vi "CSM Module - TCP Server Module(Multi-Loop Support).vi"(7 "Name(\"\" to use uuid)":string="Event CSM Tiny") -> ()   [LabVIEW 2017]
doc: "Demonstrates how to set up a basic TCP connection, send data to the specified port once a connection has been established, and terminate the connection once the data has been sent. This VI is designed to stop if the TCP connection is terminated. The data sent in this example is an array of random numbers."
uses:
  user.lib/_NEVSTOP/Communicable State Machine(CSM)/AdvanceAPI/CSM - Make String Arguments Safe.vi
  user.lib/_NEVSTOP/Communicable State Machine(CSM)/AdvanceAPI/CSM - Break Down Multiple States String.vi
  user.lib/_NEVSTOP/Communicable State Machine(CSM)/AdvanceAPI/CSM - Compact Multiple States.vi
  user.lib/_NEVSTOP/Communicable State Machine(CSM)/AdvanceAPI/CSM - Keywords.vi
  user.lib/_NEVSTOP/Communicable State Machine(CSM)/AdvanceAPI/CSM - List Modules.vi
  user.lib/_NEVSTOP/Communicable State Machine(CSM)/Communicable State Machine.lvlib
panel:
  in  "Send String":string
  out "Connected":bool
  out "TCP Received":string
  out "TCP":refnum<k5>
  out "State History":string
  # "Overview:\n\nThe sentence after polishing: \"This example demonstrates how to create a CSM module with a side loop. In some scenarios, it is much simpler to implement logic outside the CSM loop. In these cases, you can utilize the side-loop support APIs to integrate your logic with the CSM loop and form a submodule. \n\nA simple TCP server submodule is created in this example, which is intuitive and takes advantage of CSM as the interface.\n\nInstructions::\n\n1. Run this VI.\n2. Run the slightly modified Simple TCP - Client.vi, which is based on the LabVIEW example.\n3. Modify the String control on both this front panel and the client, and observe the log information.\n4. You can restart Simple TCP - Client.vi to view the logs."
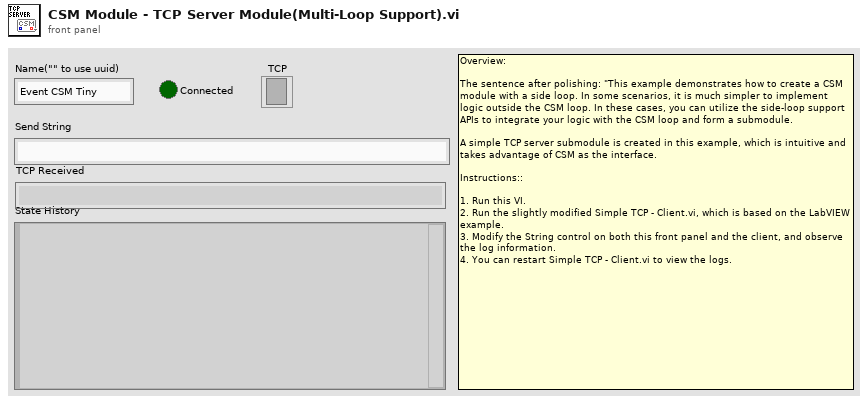
[diagram p1: front panel]
types:
  T1 = enum32{"Invalid", "Standard", "Closed", "Hidden", "Minimized", "Maximized"}
  T2 = enum32{"invalid app kind", "Development System", "Run Time System", "Student Edition", "Embedded LabVIEW", "Evaluation", "Custom"}
  T3 = typedef "Communicable State Machine.lvlib/_CSM_Response Source Message.ctl" = cluster{"‘State":string, "’Arguments":string, "’Error":errorcluster}
  T4 = cluster{"Current VI Reference":refnum<vi>, "Close Panel on Exit?":bool}
  T5 = cluster{"Core":cluster{"Current VI Reference":refnum<vi>, "Close Panel on Exit?":bool}, "Your Boolean data":bool, "Your string data":string}
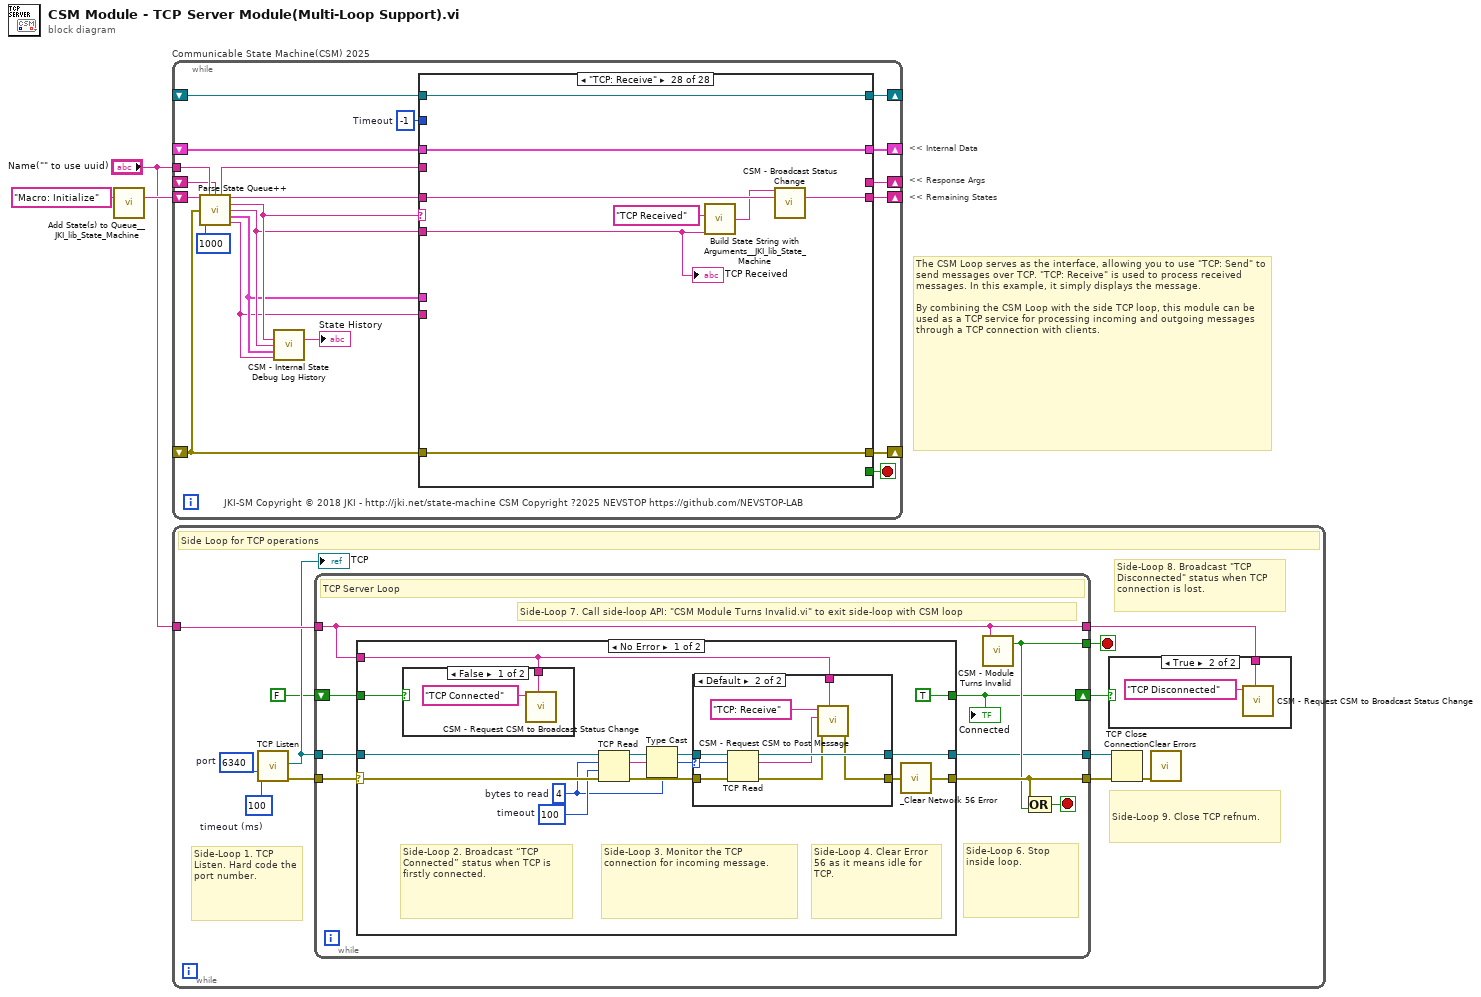
[diagram p0: block diagram]
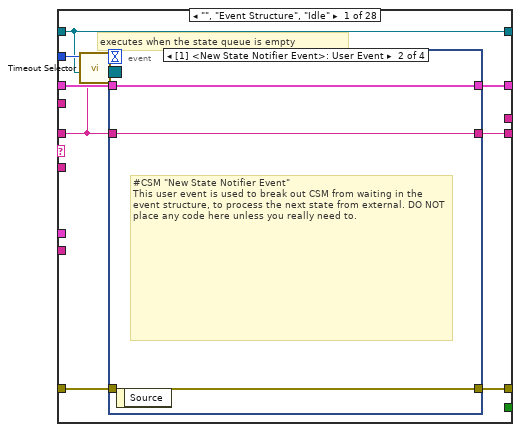
[diagram p2: hidden frame]
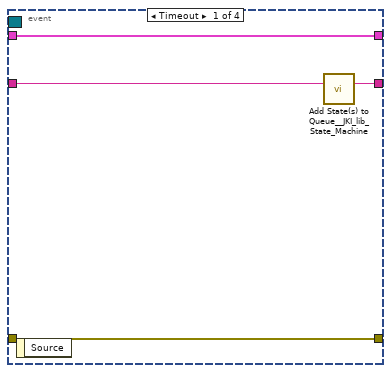
[diagram p3: hidden frame]
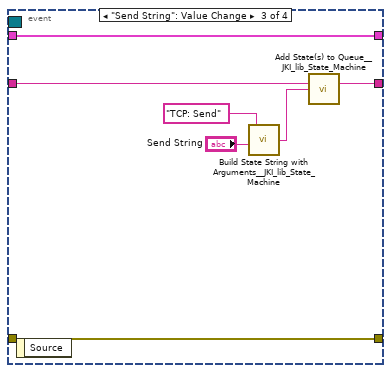
[diagram p4: hidden frame]
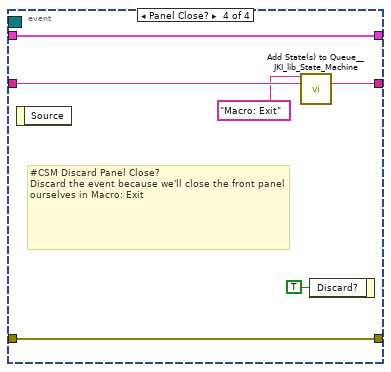
[diagram p5: hidden frame]
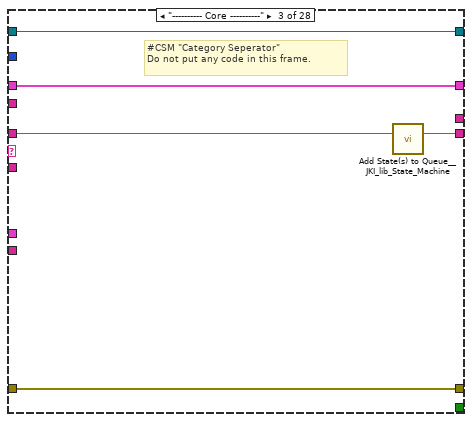
[diagram p7: hidden frame]
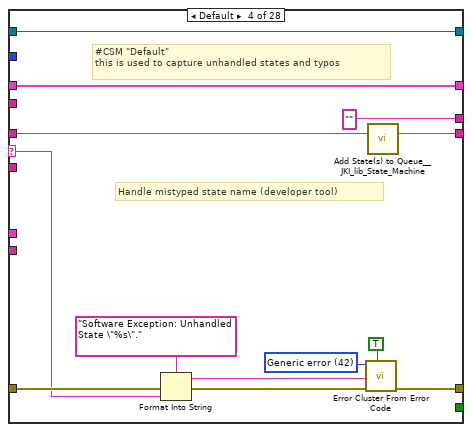
[diagram p8: hidden frame]
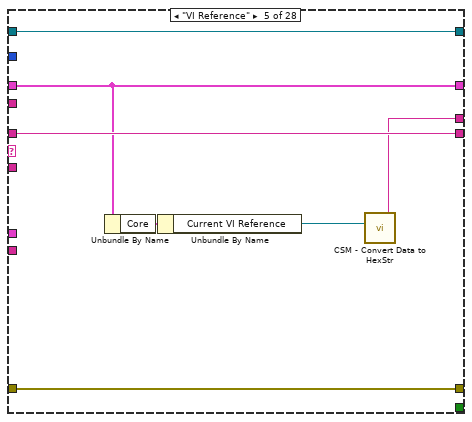
[diagram p9: hidden frame]
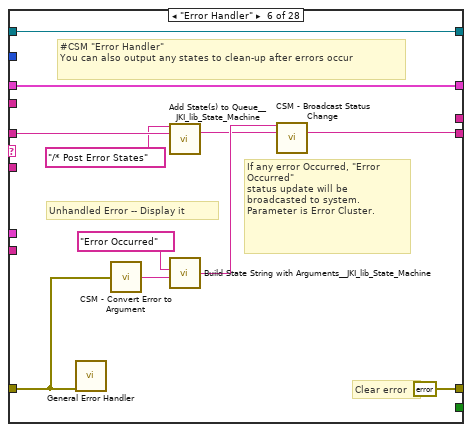
[diagram p10: hidden frame]
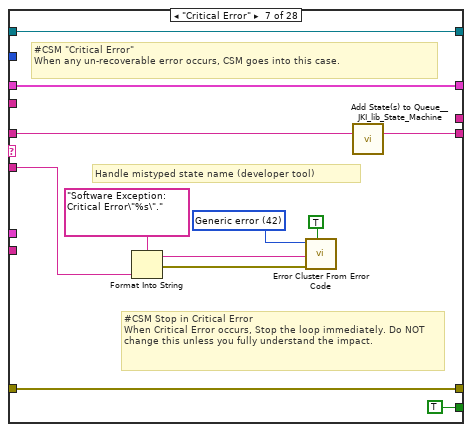
[diagram p11: hidden frame]
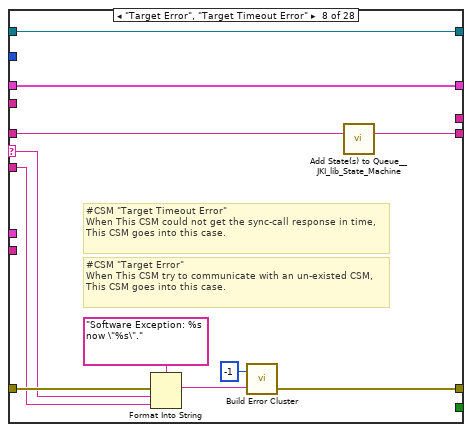
[diagram p12: hidden frame]
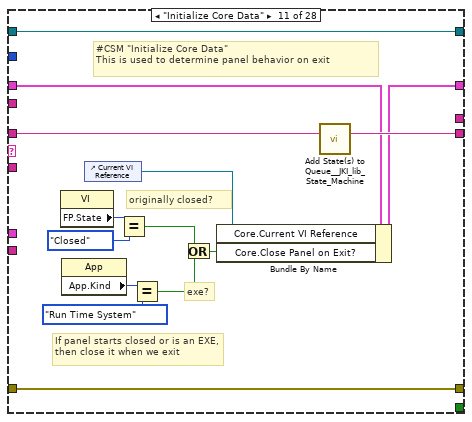
[diagram p15: hidden frame]
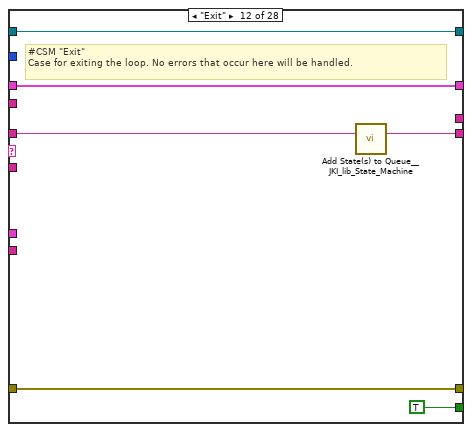
[diagram p16: hidden frame]
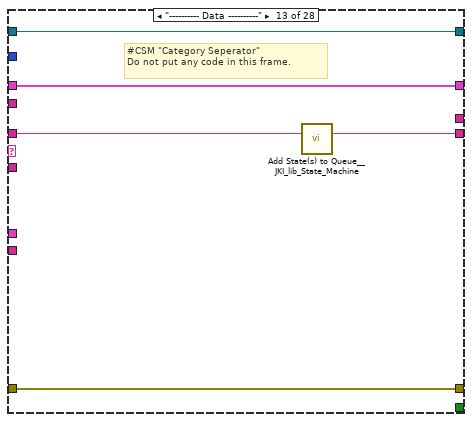
[diagram p17: hidden frame]
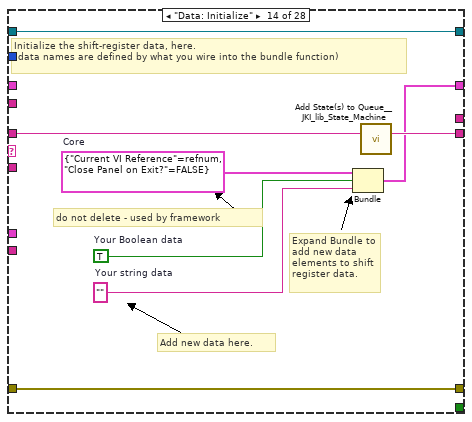
[diagram p18: hidden frame]
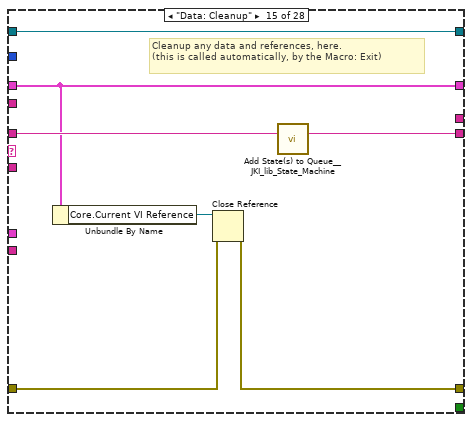
[diagram p19: hidden frame]
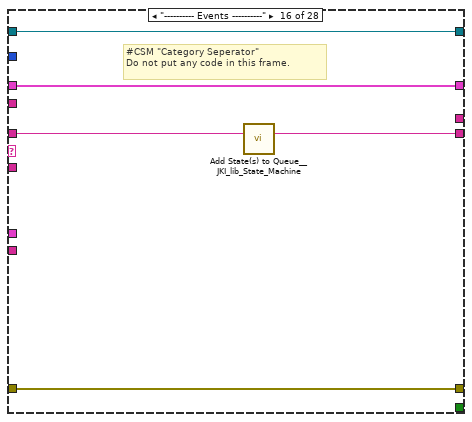
[diagram p20: hidden frame]
diagram:
  # "The CSM Loop serves as the interface, allowing you to use \"TCP: Send\" to send messages over TCP. \"TCP: Receive\" is used to process received messages. In this example, it simply displays the message. \n\nBy combining the CSM Loop with the side TCP loop, this module can be used as a TCP service for processing incoming and outgoing messages through a TCP connection with clients."
  # "<< Internal Data"
  # "<< Response Args"
  # "<< Remaining States"
  n1 = call <vilib>:"Add State(s) to Queue__JKI_lib_State_Machine.vi"("State(s) in (\"\")"="Macro: Initialize") -> ("States Out"=w2:string)  [unwired: 14 in]
  n2 = while "Communicable State Machine(CSM) 2025" {
    shift-right: [w19] -> _
    shift-left: _ -> [w18]
    shift-right: [w22] -> _
    shift-left: _ -> [w16]
    shift-right: [w21] -> _
    shift-left: w2 -> [w23]
    tunnel: "Name(\"\" to use uuid)" -> [w11]
    shift-right: [w14] -> _
    shift-left: _ -> [w5]
    shift-right: [w13] -> _
    shift-left: _ -> [w12]
    stop <- w20 stop-if-true
    w17 = -1  # Timeout
    # "JKI-SM Copyright © 2018 JKI - http://jki.net/state-machine CSM Copyright ?2025 NEVSTOP https://github.com/NEVSTOP-LAB"
    n3 = call "Parse State Queue++.vi"("State Queue"=w23, "Name(\"\" to use uuid)"=w11, "Response Arguments"=w5, "Previous Error"=w16, "Response Timeout(-2 use global Settings)"=1000 ("Response Timeout(1000ms)")) -> ("Name Used"=w6:string, "Remaining States"=w24:string, "Current State"=w10:string, "Arguments"=w9:string, ">> Response Source Message >>"=w8:T3, ">> Source CSM >>"=w7:string)  [unwired: 5 in]
    n4 = call "CSM - Internal State Debug Log History.vi"("State"=w10, "Arguments (\"\")"=w9, ">> Response Source Message >>"=w8, "Source (\"\")"=w7) -> ("Debug Log"=→"State History":string)  [unwired: 11 in]
    n5 = case shown="\"TCP: Receive\"" w10 {
      selector: w10 -> [_ _ _ w65 _ _ _ w109 _ _ _ _ _ _ _ _ _ _ _ _ _ _ _ _ _ _ _ _]
      tunnel: w24 -> [w25 w56 w62 w69 w81 w93 w103 w111 w119 w123 w138 w144 w149 w157 w164 w169 w176 w180 w186 w191 w198 w214 w284 w290 w301 w304 w315 w322]
      tunnel: w9 -> [_ _ _ _ _ _ w96 w110 _ _ _ _ _ _ _ _ _ _ _ _ w193 w208 _ _ _ _ w306 w317]
      tunnel: w18 -> [w32 w55 w59 w67 w80 w91 w104 w113 w118 w122 w131 w142 w146 _ w159 w166 w175 w179 w183 w189 w196 w210 w281 w287 w298 w303 w314 w321]
      tunnel: [w31 w57 w60 w71 w82 errorcluster {"status"=FALSE, "code"=0, "source"=""} ("error out") w105 w107 w120 w124 w135 w141 w147 w154 w160 w167 w170 w178 w184 w188 w194 w211 w282 w288 w299 w305 w307 w323] -> w22
      tunnel: w16 -> [w30 w57 w60 w70 w82 w83 w105 w115 w120 w124 w135 w141 w147 w154 w161 w167 _ w181 w184 w188 w195 w212 w282 w288 w299 w305 _ w323]
      tunnel: [w33 w56 w61 w68 w81 w84 w102 w114 w119 w123 w137 w143 w148 w156 w163 w168 w176 w180 w185 w190 w197 w213 w283 w289 w300 w304 w315 w319] -> w21
      tunnel: [_ _ _ _ _ _ TRUE _ _ _ _ TRUE _ _ _ _ _ _ _ _ _ _ _ _ _ _ _ _] -> w20
      tunnel: [w29 w55 w59 w67 w80 w91 w104 w113 w118 w122 w136 w142 w146 w155 w159 w166 w175 w179 w183 w189 w196 w210 w281 w287 w298 w303 w314 w321] -> w19
      tunnel: w17 -> [w28 _ _ _ _ _ _ _ _ _ _ _ _ _ _ _ _ _ _ _ _ _ _ _ _ _ _ _]
      tunnel: w7 -> [_ _ _ _ _ _ _ _ _ _ _ _ _ _ _ _ _ _ _ _ _ _ _ _ _ _ _ _]
      tunnel: w8 -> [_ _ _ _ _ _ _ _ _ _ _ _ _ _ _ _ _ _ _ _ _ _ _ _ _ _ _ _]
      tunnel: [_ _ _ "" w76 _ _ _ _ _ _ _ _ _ _ _ _ _ _ _ _ _ _ _ _ _ _ _] -> w14
      tunnel: [w27 w54 w58 w63 w79 w89 w94 w112 w117 w121 w125 w139 w145 w150 w158 w165 w174 w177 w182 w187 w192 w207 w280 w285 w291 w302 w313 w320] -> w13
      tunnel: w12 -> [w27 w54 w58 w63 w79 w89 w94 w112 w117 w121 w125 w139 w145 w150 w158 w165 _ w177 w182 w187 w192 w207 w280 w285 w291 w302 w313 w320]
      tunnel: w6 -> [_ _ _ _ _ _ _ _ _ _ _ _ _ _ _ _ w173 _ _ _ _ _ _ _ _ _ _ _]
      frame "", "Event Structure", "Idle" {
        # "executes when the state queue is empty"
        n6 = call "Timeout Selector.vi"("Remaining States"=w25, "Timeout Expected"=w28) -> ("Timeout"=w26:i32)  [unwired: 5 in]
        n7 = event shown="[1] <New State Notifier Event>: User Event" {
          selector: w27 -> [_ _ _ _]
          dyn-events: _ -> [_ _ _ _]
          timeout: w26 -> [_ _ _ _]
          tunnel: w25 -> [w37 w39 w45 w53]
          tunnel: [w36 w39 w44 w52] -> w33
          tunnel: w32 -> [w34 w40 w46 w50]
          tunnel: [w35 w38 w47 w51] -> w31
          tunnel: w30 -> [w35 w38 w47 w51]
          tunnel: [w34 w40 w46 w50] -> w29
          event Timeout {
            n8 = event-data() -> ()  [unwired: 1 in, 1 out]
            n9 = call <vilib>:"Add State(s) to Queue__JKI_lib_State_Machine.vi"("State(s) in (\"\")"=w37) -> ("States Out"=w36:string)  [unwired: 14 in]
          }
          event User Event {
            # "#CSM \"New State Notifier Event\"\nThis user event is used to break out CSM from waiting in the event structure, to process the next state from external. DO NOT place any code here unless you really need to."
            n10 = event-data() -> ()  [unwired: 1 in, 1 out]
          }
          event "Send String": Value Change {
            n11 = event-data() -> ()  [unwired: 1 in, 1 out]
            n12 = call <vilib>:"Build State String with Arguments__JKI_lib_State_Machine.vi"("Arguments (\"\")"="Send String", "State"="TCP: Send") -> ("State with Arguments"=w42:string)  [unwired: 4 in]
            n13 = call <vilib>:"Add State(s) to Queue__JKI_lib_State_Machine.vi"("State(s) in (\"\")"=w45, "State(s) at Back (\"\")"=w42) -> ("States Out"=w44:string)  [unwired: 13 in]
          }
          event Panel Close? {
            # "#CSM Discard Panel Close?\nDiscard the event because we'll close the front panel ourselves in Macro: Exit"
            n14 = event-data() -> ()  [unwired: 1 in, 1 out]
            n15 = call <vilib>:"Add State(s) to Queue__JKI_lib_State_Machine.vi"("State(s) in Front (\"\")"="Macro: Exit", "State(s) in (\"\")"=w53) -> ("States Out"=w52:string)  [unwired: 13 in]
            n16 = event-data("Discard?"=TRUE) -> ()  [unwired: 1 in, 1 out]
          }
        }
      }
      frame "CSM Documentation" {
        # "#CSM README FIRST\n\nCSM is a LabVIEW application framework that builds upon JKI State Machine (JKISM). It follows the pattern of JKISM and extends the keywords to describe message communication between CSM modules, including concepts such as Sync-Message, Async-Message, Subscription/Unsubscription of status - essential elements for creating reusable code modules. For more information, please visit the CSM wiki: https://github.com/NEVSTOP-LAB/JKI-State-Machine-Plus-Plus/wiki\n\nFor instructions on JKI State Machine, visit: http://jki.net/state-machine/\nFor information about CSM, visit: https://github.com/NEVSTOP-LAB"
        # "#CSM \"Documentation\"\nCase for holding CSM Documenation"
      }
      frame "---------- Core ----------" {
        # "#CSM \"Category Seperator\"\nDo not put any code in this frame."
        n17 = call <vilib>:"Add State(s) to Queue__JKI_lib_State_Machine.vi"("State(s) in (\"\")"=w62) -> ("States Out"=w61:string)  [unwired: 14 in]
      }
      frame Default {
        w74 = 42 items=["No error", "Argument error", "Memory is full", "Out of zone", "End of file", "File already open", "Generic file I/O error", "File not found", "File permission error", "Disk is full", "Duplicate path", "Too many files open", "System feature not enabled", "Resource file not found", "Cannot add resource", "Resource not found", "Image not found", "Image memory error", "Pen does not exist", "Config type invalid", "Config token not found", "Config parse error", "Config memory error", "Bad external code format", "Bad external code offset", "External code not present", "Null window", "Destroy window error", "Null menu", "Print aborted", "Bad print record", "Print driver error", "Windows error during printing", "Memory error during printing", "Print dialog error", "Generic print error", "Invalid device refnum", "Device not found", "Device parameter error", "Device unit error", "Cannot open device", "Device call aborted", "Generic error", "Cancelled by user", "Object ID too low", "Object ID too high", "Object not in heap", "Unknown heap", "Unknown object (invalid DefProc)", "Unknown object (DefProc not in table)", "Message out of range", "Invalid (null) method", "Unknown message", "Manager call not supported", "Bad address", "Network operation in progress", "Network operation timed out", "Connection is busy", "Network attribute not supported", "Network error", "Address in use", "System out of memory", "Connection aborted", "Connection refused", "Not connected", "Already connected", "Connection closed", "Initialization error (interapplication manager)", "Bad occurrence", "Wait on unbound occurrence handler", "Occurrence queue overflow", "Datalog type conflict", "Unused", "Unrecognized type (interapplication manager)", "Memory corrupt", "Failed to make temporary DLL", "Old CIN version", "Drag socket not found", "Failed to load drop-object", "Failed to register OLE object", "Failed to release OLE object", "Format specifier type mismatch", "Unknown format specifier", "Too few format specifiers", "Too many format specifiers", "Scan failed", "Newer CIN version", "Error converting to variant", "Runtime menu error", "Password tampered", "Variant attribute not found", "Incompatible variant data type", "Event data is not available", "Event Store is not present", "Occurrence is not found", "Event Queue is not created", "Event info is not available", "Refnum passed is NULL", "Error retrieving Class GUID", "Error retrieving CoClass GUID", "Error retrieving TypeLib GUID.", "Bad built application magic bytes.", "Specific driver is different from the specific driver associated with the Logical Name.", "There is no session opened to the class driver.", "Max Error", "MAX - Error with config objects", "MAX - Error loading configuration", "MAX - Group not supported"]
        # "#CSM \"Default\"\nthis is used to capture unhandled states and typos"
        # "Handle mistyped state name (developer tool)"
        n18 = Format Into String(format string="Software Exception: Unhandled State \"%s\"." ("message"), error in=w70, w65) -> (resulting string=w73:string, error out=w72:errorcluster)  [unwired: 1 in]
        n19 = call <vilib>:"Error Cluster From Error Code.vi"("show call chain? (False)"=TRUE, "error in (no error)"=w72, "error message (\"\")"=w73, "error code (0)"=w74) -> ("error out"=w71:errorcluster)  [unwired: 5 in]
        n20 = call <vilib>:"Add State(s) to Queue__JKI_lib_State_Machine.vi"("State(s) in (\"\")"=w69) -> ("States Out"=w68:string)  [unwired: 14 in]
      }
      frame "VI Reference" {
        n21 = Unbundle By Name(w80) -> ("Core"=w78:T4)
        n22 = Unbundle By Name(w78) -> ("Current VI Reference"=w77:refnum<vi>)
        n23 = call "CSM - Convert Data to HexStr.vi"("Variant"=w77) -> ("HEX String (0-9,A-F)"=w76:string)  [unwired: 8 in]
      }
      frame "Error Handler" {
        # "#CSM \"Error Handler\"\nYou can also output any states to clean-up after errors occur"
        # "If any error Occurred, \"Error Occurred\" \nstatus update will be broadcasted to system.\nParameter is Error Cluster."
        # "Unhandled Error -- Display it"
        # "Clear error"
        n24 = call <vilib>:"General Error Handler.vi"("error in (no error)"=w83) -> ()  [unwired: 10 in, 5 out]
        n25 = call "CSM - Convert Error to Argument.vi"("error"=w83) -> ("Argument"=w87:string)  [unwired: 4 in]
        n26 = call <vilib>:"Add State(s) to Queue__JKI_lib_State_Machine.vi"("State(s) in Front (\"\")"="/* Post Error States", "State(s) in (\"\")"=w93) -> ("States Out"=w85:string)  [unwired: 13 in]
        n27 = call <vilib>:"Build State String with Arguments__JKI_lib_State_Machine.vi"("Arguments (\"\")"=w87, "State"="Error Occurred" ("Status with Arguments")) -> ("State with Arguments"=w86:string)  [unwired: 4 in]
        n28 = call "CSM - Broadcast Status Change.vi"("Status with Arguments"=w86, "State Queue"=w85) -> ("Remaining States"=w84:string)  [unwired: 13 in]
      }
      frame "Critical Error" {
        w100 = 42 items=["No error", "Argument error", "Memory is full", "Out of zone", "End of file", "File already open", "Generic file I/O error", "File not found", "File permission error", "Disk is full", "Duplicate path", "Too many files open", "System feature not enabled", "Resource file not found", "Cannot add resource", "Resource not found", "Image not found", "Image memory error", "Pen does not exist", "Config type invalid", "Config token not found", "Config parse error", "Config memory error", "Bad external code format", "Bad external code offset", "External code not present", "Null window", "Destroy window error", "Null menu", "Print aborted", "Bad print record", "Print driver error", "Windows error during printing", "Memory error during printing", "Print dialog error", "Generic print error", "Invalid device refnum", "Device not found", "Device parameter error", "Device unit error", "Cannot open device", "Device call aborted", "Generic error", "Cancelled by user", "Object ID too low", "Object ID too high", "Object not in heap", "Unknown heap", "Unknown object (invalid DefProc)", "Unknown object (DefProc not in table)", "Message out of range", "Invalid (null) method", "Unknown message", "Manager call not supported", "Bad address", "Network operation in progress", "Network operation timed out", "Connection is busy", "Network attribute not supported", "Network error", "Address in use", "System out of memory", "Connection aborted", "Connection refused", "Not connected", "Already connected", "Connection closed", "Initialization error (interapplication manager)", "Bad occurrence", "Wait on unbound occurrence handler", "Occurrence queue overflow", "Datalog type conflict", "Unused", "Unrecognized type (interapplication manager)", "Memory corrupt", "Failed to make temporary DLL", "Old CIN version", "Drag socket not found", "Failed to load drop-object", "Failed to register OLE object", "Failed to release OLE object", "Format specifier type mismatch", "Unknown format specifier", "Too few format specifiers", "Too many format specifiers", "Scan failed", "Newer CIN version", "Error converting to variant", "Runtime menu error", "Password tampered", "Variant attribute not found", "Incompatible variant data type", "Event data is not available", "Event Store is not present", "Occurrence is not found", "Event Queue is not created", "Event info is not available", "Refnum passed is NULL", "Error retrieving Class GUID", "Error retrieving CoClass GUID", "Error retrieving TypeLib GUID.", "Bad built application magic bytes.", "Specific driver is different from the specific driver associated with the Logical Name.", "There is no session opened to the class driver.", "Max Error", "MAX - Error with config objects", "MAX - Error loading configuration", "MAX - Group not supported"]
        # "#CSM Stop in Critical Error\nWhen Critical Error occurs, Stop the loop immediately. Do NOT change this unless you fully understand the impact."
        # "#CSM \"Critical Error\"\nWhen any un-recoverable error occurs, CSM goes into this case."
        # "Handle mistyped state name (developer tool)"
        n29 = Format Into String(format string="Software Exception: Critical Error\"%s\"." ("message"), w96) -> (resulting string=w99:string, error out=w98:errorcluster)  [unwired: 2 in]
        n30 = call <vilib>:"Error Cluster From Error Code.vi"("show call chain? (False)"=TRUE, "error in (no error)"=w98, "error message (\"\")"=w99, "error code (0)"=w100) -> ()  [unwired: 5 in, 1 out]
        n31 = call <vilib>:"Add State(s) to Queue__JKI_lib_State_Machine.vi"("State(s) in (\"\")"=w103) -> ("States Out"=w102:string)  [unwired: 14 in]
      }
      frame "Target Error", "Target Timeout Error" {
        # "#CSM \"Target Error\"\nWhen This CSM try to communicate with an un-existed CSM, This CSM goes into this case."
        # "#CSM \"Target Timeout Error\"\nWhen This CSM could not get the sync-call response in time, This CSM goes into this case."
        n32 = Format Into String(format string="Software Exception: %s now \"%s\"." ("message"), error in=w115, w109, w110) -> (resulting string=w108:string)  [unwired: 1 in, 1 out]
        n33 = call "Build Error Cluster.vi"("String to Prepend to source (\"\")"=w108, "code"=-1) -> ("error out"=w107:errorcluster)
        n34 = call <vilib>:"Add State(s) to Queue__JKI_lib_State_Machine.vi"("State(s) in (\"\")"=w111) -> ("States Out"=w114:string)  [unwired: 14 in]
      }
      frame "Async Response", "Response" {
        # "#CSM Response Comments\nAfter Message is executed, CSM goes to this state for receive the response.\n    For Async Message(->), \"Async Response\" is used. This CSM will goes to \"Async Message Posted\" immediately and receive the \"Async Response\" after the callee finishes the message.\n    For Sync Message(@),  This CSM will wait until the message is done and immediately goes to \"Response\""
        # "#CSM \"Async Response\"\nHandle Async-call Response (\"Async Response\" for ->)"
        # "#CSM \"Response\"\nHandle Sync-call Response (\"Response\" for -@)"
      }
      frame "Async Message Posted" {
        # "#CSM \"Async Message Posted\"\nAfter Async Message is posted (-> or ->| ), CSM goes to this state for post-action.\nYou can use Argument - State to tell which Async Message is called."
      }
      frame "Initialize Core Data" {
        # "#CSM \"Initialize Core Data\"\nThis is used to determine panel behavior on exit"
        # "originally closed?"
        # "exe?"
        # "If panel starts closed or is an EXE, then close it when we exit"
        n35 = property class="VI"() -> ("FP.State"=w128:T1)  [unwired: 2 in, 2 out]
        n36 = property class="App"() -> ("App.Kind"=w134:T2)  [unwired: 2 in, 2 out]
        n37 = control-ref of="Current VI Reference"() -> (w129:refnum<vi>)
        n38 = Equal?(x=w128, y=T1."Closed" ("Front Panel Window:State")) -> (x = y?=w126:bool)
        n39 = Equal?(x=w134, y=T2."Run Time System" ("Application:Kind")) -> (x = y?=w132:bool)
        n40 = Or(x=w126, y=w132) -> (x .or. y?=w130:bool)
        n41 = Bundle By Name(cluster=w131, "Core.Current VI Reference"=w129, "Core.Close Panel on Exit?"=w130) -> (w136:T5)
        n42 = call <vilib>:"Add State(s) to Queue__JKI_lib_State_Machine.vi"("State(s) in (\"\")"=w138) -> ("States Out"=w137:string)  [unwired: 14 in]
      }
      frame "Exit" {
        # "#CSM \"Exit\"\nCase for exiting the loop. No errors that occur here will be handled."
        n43 = call <vilib>:"Add State(s) to Queue__JKI_lib_State_Machine.vi"("State(s) in (\"\")"=w144) -> ("States Out"=w143:string)  [unwired: 14 in]
      }
      frame "---------- Data ----------" {
        # "#CSM \"Category Seperator\"\nDo not put any code in this frame."
        n44 = call <vilib>:"Add State(s) to Queue__JKI_lib_State_Machine.vi"("State(s) in (\"\")"=w149) -> ("States Out"=w148:string)  [unwired: 14 in]
      }
      frame "Data: Initialize" {
        w151 = T4 {"Current VI Reference"=refnum, "Close Panel on Exit?"=FALSE}  # Core
        w153 = TRUE  # Your Boolean data
        w152 = ""  # Your string data
        # "do not delete - used by framework"
        # "Expand Bundle to add new data elements to shift register data."
        # "Add new data here."
        # "Initialize the shift-register data, here.\n(data names are defined by what you wire into the bundle function)"
        n45 = Bundle("Core"=w151, "Your Boolean data"=w153, "Your string data"=w152) -> (w155:T5)  [unwired: 1 in]
        n46 = call <vilib>:"Add State(s) to Queue__JKI_lib_State_Machine.vi"("State(s) in (\"\")"=w157) -> ("States Out"=w156:string)  [unwired: 14 in]
      }
      frame "Data: Cleanup" {
        # "Cleanup any data and references, here.\n(this is called automatically, by the Macro: Exit)"
        n47 = Unbundle By Name(w159) -> ("Core.Current VI Reference"=w162:refnum<vi>)
        n48 = Close Reference(reference=w162, error in (no error)=w161) -> (error out=w160:errorcluster)
        n49 = call <vilib>:"Add State(s) to Queue__JKI_lib_State_Machine.vi"("State(s) in (\"\")"=w164) -> ("States Out"=w163:string)  [unwired: 14 in]
      }
      frame "---------- Events ----------" {
        # "#CSM \"Category Seperator\"\nDo not put any code in this frame."
        n50 = call <vilib>:"Add State(s) to Queue__JKI_lib_State_Machine.vi"("State(s) in (\"\")"=w169) -> ("States Out"=w168:string)  [unwired: 14 in]
      }
      frame "Events: Register" {
        # "#CSM \"Events: Register\"\nRegister user event. New Message Event is registered to break CSM waiting in event structure by default."
        # "#CSM Register New Message Event\nRegister message event to break Waiting in Event structure."
        n51 = call "CSM - Get New State Notifier Event.vi"("Name(\"\" to use uuid) in"=w173) -> ("Error out"=w171:errorcluster, "New State Notifier Event"=w172:refnum<user-event>)  [unwired: 9 in]
        n52 = register-events(error in=w171, w172) -> (reference out=w174:refnum<event-registration>, error out=w170:errorcluster)  [unwired: 1 in]
      }
      frame "Events: Unregister" {
        # "#CSM \"Events: Unregister\"\nUnregister user event."
        n53 = Unregister For Events(event registration refnum=w177, error in=w181) -> (error out=w178:errorcluster)
      }
      frame "---------- UI ----------" {
        # "#CSM \"Category Seperator\"\nDo not put any code in this frame."
        n54 = call <vilib>:"Add State(s) to Queue__JKI_lib_State_Machine.vi"("State(s) in (\"\")"=w186) -> ("States Out"=w185:string)  [unwired: 14 in]
      }
      frame "UI: Initialize" {
        # "#CSM \"UI: Initialize\"\nInitialize the User Interface, here.\n(this is called automatically, by the Macro: Init)"
        n55 = call <vilib>:"Add State(s) to Queue__JKI_lib_State_Machine.vi"("State(s) in (\"\")"=w191) -> ("States Out"=w190:string)  [unwired: 14 in]
      }
      frame "UI: Cursor Set" {
        # "#CSM \"UI: Cursor Set\"\nSet and Unset Cursor Busy.\n(Usage: \"UI: Cursor Set >> Busy|Idle\")"
        # "Argument"
        n56 = disable-structure shown="TARGET_TYPE!=Windows" {
          disable-tunnel: w195 -> [w201 w206]
          disable-tunnel: [w200 w206] -> w194
          disable-tunnel: w193 -> [w199 _]
          frame condition #0 (active) {
            n57 = case shown="\"Idle\", Default" w199 {
              tunnel: w201 -> [w203 w205]
              tunnel: [w202 w204] -> w200
              frame "Idle", Default {
                n58 = call <vilib>:"Unset Busy.vi"("error in (no error)"=w203) -> ("error out"=w202:errorcluster)  [unwired: 10 in]
              }
              frame "Busy" {
                n59 = call <vilib>:"Set Busy.vi"("error in (no error)"=w205) -> ("error out"=w204:errorcluster)  [unwired: 9 in, 1 out]
              }
            }
          }
          frame condition #1 {
          }
        }
        n60 = call <vilib>:"Add State(s) to Queue__JKI_lib_State_Machine.vi"("State(s) in (\"\")"=w198) -> ("States Out"=w197:string)  [unwired: 14 in]
      }
      frame "UI: Front Panel State" {
        # "#CSM \"UI: Front Panel State\"\nSet Front Panel Open or Closed\n(Usage: \"UI: Front Panel State >> Open|Close\")"
        # "Argument"
        n61 = Unbundle By Name(w210) -> ("Core.Current VI Reference"=w209:refnum<vi>)
        n62 = call <vilib>:"Add State(s) to Queue__JKI_lib_State_Machine.vi"("State(s) in (\"\")"=w214) -> ("States Out"=w213:string)  [unwired: 14 in]
        n63 = case shown="\"Close\", \"Closed\"" w208 {
          tunnel: w212 -> [w220 w235 w246 w259 w272]
          tunnel: [w222 w236 w248 w261 w274] -> w211
          tunnel: w209 -> [w221 w233 w247 w260 w273]
          frame "Open", "Standard", Default {
            w215 = T1."Standard" ("State")
            n64 = property class="VI"(reference=w221, error in=w220) -> (reference out=w218:refnum<vi>, error out=w219:errorcluster, "FP.State"=w217:T1)
            n65 = Not Equal?(x=w217, y=w215) -> (x != y?=w216:bool)
            n66 = case shown="True" w216 {
              tunnel: [w226 w228] -> w222
              tunnel: w219 -> [w225 w228]
              tunnel: w218 -> [w224 _]
              tunnel: w215 -> [w223 _]
              frame True {
                n67 = invoke class="VI" method="FP.Open"(reference=w224, error in=w225, "Activate"=TRUE, "State"=w223) -> (error out=w226:errorcluster)  [unwired: 1 in, 4 out]
              }
              frame False {
              }
            }
          }
          frame "Close", "Closed" {
            n68 = property class="VI"(reference=w233, error in=w235) -> (reference out=w232:refnum<vi>, error out=w234:errorcluster, "FP.State"=w230:T1)
            n69 = Not Equal?(x=w230, y=T1."Closed" ("Front Panel Window:State")) -> (x != y?=w229:bool)
            n70 = case shown="False" w229 {
              tunnel: [w237 w240] -> w236
              tunnel: w234 -> [w237 w239]
              tunnel: w232 -> [_ w238]
              frame False {
              }
              frame True {
                n71 = invoke class="VI" method="FP.Close"(reference=w238, error in=w239) -> (error out=w240:errorcluster)  [unwired: 1 in, 2 out]
              }
            }
          }
          frame "Hidden", "Hide" {
            w241 = T1."Hidden" ("State")
            n72 = property class="VI"(reference=w247, error in=w246) -> (reference out=w244:refnum<vi>, error out=w245:errorcluster, "FP.State"=w243:T1)
            n73 = Not Equal?(x=w243, y=w241) -> (x != y?=w242:bool)
            n74 = case shown="True" w242 {
              tunnel: [w252 w253] -> w248
              tunnel: w245 -> [w251 w253]
              tunnel: w244 -> [w250 _]
              tunnel: w241 -> [w249 _]
              frame True {
                n75 = invoke class="VI" method="FP.Open"(reference=w250, error in=w251, "State"=w249) -> (error out=w252:errorcluster)  [unwired: 2 in, 4 out]
              }
              frame False {
              }
            }
          }
          frame "Minimize", "Minimized" {
            w254 = T1."Minimized" ("State")
            n76 = property class="VI"(reference=w260, error in=w259) -> (reference out=w257:refnum<vi>, error out=w258:errorcluster, "FP.State"=w256:T1)
            n77 = Not Equal?(x=w256, y=w254) -> (x != y?=w255:bool)
            n78 = case shown="True" w255 {
              tunnel: [w265 w266] -> w261
              tunnel: w258 -> [w264 w266]
              tunnel: w257 -> [w263 _]
              tunnel: w254 -> [w262 _]
              frame True {
                n79 = invoke class="VI" method="FP.Open"(reference=w263, error in=w264, "State"=w262) -> (error out=w265:errorcluster)  [unwired: 2 in, 4 out]
              }
              frame False {
              }
            }
          }
          frame "Maximize", "Maximized" {
            w267 = T1."Maximized" ("State")
            n80 = property class="VI"(reference=w273, error in=w272) -> (reference out=w270:refnum<vi>, error out=w271:errorcluster, "FP.State"=w269:T1)
            n81 = Not Equal?(x=w269, y=w267) -> (x != y?=w268:bool)
            n82 = case shown="True" w268 {
              tunnel: [w278 w279] -> w274
              tunnel: w271 -> [w277 w279]
              tunnel: w270 -> [w276 _]
              tunnel: w267 -> [w275 _]
              frame True {
                n83 = invoke class="VI" method="FP.Open"(reference=w276, error in=w277, "State"=w275) -> (error out=w278:errorcluster)  [unwired: 2 in, 4 out]
              }
              frame False {
              }
            }
          }
        }
      }
      frame "---------- Macro ----------" {
        # "#CSM \"Category Seperator\"\nDo not put any code in this frame."
        n84 = call <vilib>:"Add State(s) to Queue__JKI_lib_State_Machine.vi"("State(s) in (\"\")"=w284) -> ("States Out"=w283:string)  [unwired: 14 in]
      }
      frame "Macro: Initialize" {
        w286 = "Data: Initialize\nInitialize Core Data\nEvents: Register\nUI: Initialize\n//UI: Front Panel State >> Open"  # Data: Initialize Initialize Core Data Events: Register UI: Initialize //UI: Front Panel State >> Open
        # "#CSM \"Macro: Initialize\"\nInitialization Macro (This is called once, when the VI starts)"
        n85 = call <vilib>:"Add State(s) to Queue__JKI_lib_State_Machine.vi"("State(s) in Front (\"\")"=w286, "State(s) in (\"\")"=w290) -> ("States Out"=w289:string)  [unwired: 13 in]
      }
      frame "Macro: Exit" {
        # "#CSM \"Macro: Exit\"\nExit Macro (This is called once, when the VI exits)"
        n86 = Unbundle By Name(w298) -> ("Core.Close Panel on Exit?"=w297:bool)
        n87 = Select(t="UI: Front Panel State >> Close", s=w297, f="") -> (s? t:f=w294:string)
        n88 = call <vilib>:"Add State(s) to Queue__JKI_lib_State_Machine.vi"("State(s) in (\"\")"=w294, "State(s) at Back (\"\")"="Data: Cleanup\nEvents: Unregister\nExit") -> ("States Out"=w292:string)  [unwired: 13 in]
        n89 = call <vilib>:"Add State(s) to Queue__JKI_lib_State_Machine.vi"("State(s) in Front (\"\")"=w292, "State(s) in (\"\")"=w301) -> ("States Out"=w300:string)  [unwired: 13 in]
      }
      frame "---------- API ----------" {
        # "#CSM \"Category Seperator\"\nDo not put any code in this frame."
      }
      frame "TCP: Send" {
        n90 = local read "TCP"() -> (w308:refnum<k5>)
        n91 = String Length(string=w306) -> (length=w310:i32)
        n92 = Type Cast(x=w310) -> (*(type *) &x=w309:string)  [unwired: 1 out]
        n93 = TCP Write(connection ID=w308, data in=w309) -> (connection ID out=w312:refnum<k5>, error out=w311:errorcluster)  [unwired: 1 in, 2 out]
        n94 = TCP Write(connection ID=w312, data in=w306, error in (no error)=w311) -> (error out=w307:errorcluster)  [unwired: 3 out]
      }
      frame "TCP: Receive" {
        n95 = call <vilib>:"Build State String with Arguments__JKI_lib_State_Machine.vi"("Arguments (\"\")"=w317, "State"="TCP Received") -> ("State with Arguments"=w316:string)  [unwired: 4 in]
        n96 = call "CSM - Broadcast Status Change.vi"("Status with Arguments"=w316, "State Queue"=w322) -> ("Remaining States"=w319:string)  [unwired: 13 in]
        "TCP Received" <- w317
      }
    }
  }
  n97 = while {
    tunnel: "Name(\"\" to use uuid)" -> [w330]
    stop <- w331 stop-if-true
    w332 = u16 6340  # port
    w333 = 100  # timeout (ms)
    # "Side-Loop 9. Close TCP refnum."
    # "Side-Loop 8. Broadcast \"TCP Disconnected\" status when TCP connection is lost."
    # "Side-Loop 1. TCP Listen. Hard code the port number."
    # "Side Loop for TCP operations"
    n98 = call <vilib>:"TCP Listen.vi"("timeout ms (wait forever: -1)"=w333, "port"=w332) -> ("error out"=w334:errorcluster, "connection ID"=w329:refnum<k5>)  [unwired: 5 in, 3 out]
    "TCP" <- w329
    n99 = while {
      tunnel: [w345] -> w326
      tunnel: [w341] -> w335
      tunnel: w329 -> [w343]
      tunnel: w334 -> [w342]
      tunnel: [w344] -> w331
      tunnel: w330 -> [w339]
      tunnel: [w339] -> w327
      shift-right: [w338] -> w324
      shift-left: FALSE -> [w340]
      stop <- w346 stop-if-true
      # "Side-Loop 7. Call side-loop API: \"CSM Module Turns Invalid.vi\" to exit side-loop with CSM loop"
      # "Side-Loop 6. Stop inside loop."
      # "TCP Server Loop"
      n100 = case shown="No Error" w342 {
        selector: w342 -> [w358 w377]
        tunnel: [w360 w377] -> w345
        tunnel: w343 -> [w359 w376]
        tunnel: [w355 w376] -> w341
        tunnel: w340 -> [w349 _]
        tunnel: w339 -> [w350 _]
        tunnel: [TRUE FALSE] -> w338
        frame No Error {
          w352 = 100  # timeout
          w347 = 4  # bytes to read
          # "Side-Loop 4. Clear Error 56 as it means idle for TCP."
          # "Side-Loop 3. Monitor the TCP connection for incoming message."
          # "Side-Loop 2. Broadcast “TCP Connected” status when TCP is firstly connected."
          n101 = case shown="False" w349 {
            tunnel: w350 -> [w373 _]
            frame False {
              n102 = call "CSM - Request CSM to Broadcast Status Change.vi"("Module Name"=w373, "Status"="TCP Connected") -> ()  [unwired: 9 in, 1 out]
            }
            frame True {
            }
          }
          n103 = TCP Read(connection ID=w359, bytes to read=w347, error in (no error)=w358, 9:w352) -> (connection ID out=w356:refnum<k5>, data out=w354:string, error out=w357:errorcluster)  [unwired: 1 out]
          n104 = Type Cast(type=w347, x=w354) -> (*(type *) &x=w353:i32)
          n105 = case shown="Default" w353 {
            selector: w353 -> [_ w368]
            tunnel: w357 -> [w361 w371]
            tunnel: w356 -> [w362 w370]
            tunnel: [w362 w369] -> w355
            tunnel: [w361 w365] -> w351
            tunnel: w350 -> [_ w364]
            frame 0 {
            }
            frame Default {
              n106 = TCP Read(connection ID=w370, bytes to read=w368, error in (no error)=w371) -> (connection ID out=w369:refnum<k5>, data out=w363:string, error out=w366:errorcluster)  [unwired: 2 out]
              n107 = call "CSM - Request CSM to Post Message.vi"("Module Name"=w364, "Error In (no error)"=w366, "Arguments (\"\")"=w363, "State"="TCP: Receive") -> ("error out"=w365:errorcluster)  [unwired: 7 in]
            }
          }
          n108 = call "_Clear Network 56 Error.vi"("error in (no error)"=w351) -> ("error out"=w360:errorcluster)  [unwired: 4 in]
        }
        frame Error {
          # "Side-Loop 2. No Connection is created. Wait 100ms for reconnection"
          n109 = Wait (ms)(milliseconds to wait=u32 100) -> ()  [unwired: 1 out]
        }
      }
      "Connected" <- w338
      n110 = call "CSM - Module Turns Invalid.vi"("CSM Name"=w339) -> ("Turn Invalid(Exit)?"=w344:bool)  [unwired: 2 in]
      n111 = Compound Arithmetic op=OR(w345, w344) -> (w346:bool)
    }
    n112 = case shown="True" w324 {
      tunnel: w327 -> [_ w337]
      frame False {
      }
      frame True {
        n113 = call "CSM - Request CSM to Broadcast Status Change.vi"("Module Name"=w337, "Status"="TCP Disconnected") -> ()  [unwired: 9 in, 1 out]
      }
    }
    n114 = TCP Close Connection(connection ID=w335, error in (no error)=w326) -> (error out=w328:errorcluster)  [unwired: 2 out]
    n115 = call <vilib>:"Clear Errors.vi"("error in (no error)"=w328) -> ()  [unwired: 5 in, 2 out]
  }
